vi "Day04-01_변수3 (글로벌 변수).vi"   [LabVIEW 2021]
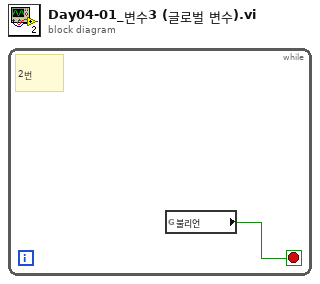
[diagram p0: block diagram]
diagram:
  n1 = while {
    stop <- w1 stop-if-true
    # "2번"
    n2 = global read "Day04-01_변수 (글로벌 변수).vi" "불리언"() -> (w1:bool)
  }
